vi "Maximize Window.vi"(8 "error in (no error)":errorcluster, 10 "window name (\"\")":string, 11 "window refnum (NaWR)":T1) -> (0 "error out":errorcluster, 3 "window refnum out":T1)   [LabVIEW 2020, in "MacroAssert.lvlib" / "WINUTIL.lvlib"]
doc: "This function will maximize the window named in the window name input, or identified by the window refnum. If an invalid window refnum is passed in, then the function will use the window name to get a window window refnum. If the window cannot be found, an error will be returned."
uses:
  WINUTIL.lvlib
  Window Refnum.ctl
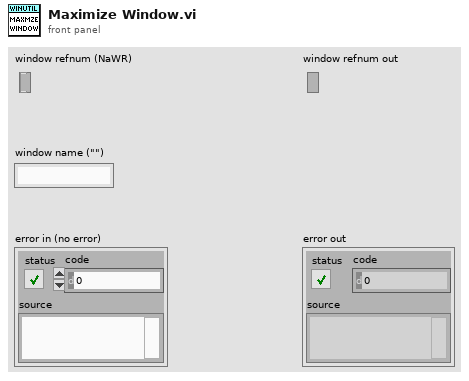
[diagram p1: front panel]
types:
  T1 = typedef "MacroAssert.lvlib/WINUTIL.lvlib/Window Refnum.ctl" = refnum<k1>
  T2 = enum8{"Maximize Window", "Minimize Window", "Show Task List", "Start Screen Saver", "Quit Application"}
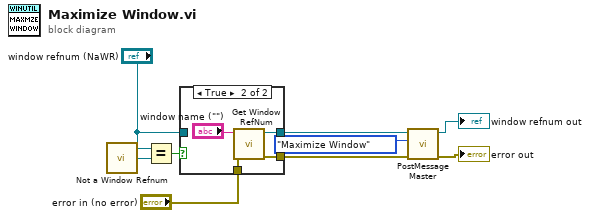
[diagram p0: block diagram]
diagram:
  n1 = call "Not a Window Refnum.vi"() -> ("Not a Window Refnum"=w7:T1)
  n2 = Equal?(x="window refnum (NaWR)", y=w7) -> (x = y?=w8:bool)
  n3 = case shown="True" w8 {
    tunnel: "error in (no error)" -> [w10 w15]
    tunnel: [w11 w14] -> w4
    tunnel: "window refnum (NaWR)" -> [w11 _]
    tunnel: [w10 w13] -> w3
    frame False {
    }
    frame True {
      n4 = call "Get Window RefNum.vi"("error in (no error)"=w15, "window name (\"\")"="window name (\"\")") -> ("error out"=w13:errorcluster, "window refnum (NaWR)"=w14:T1)  [unwired: 8 in]
    }
  }
  n5 = call "PostMessage Master.vi"("error in (no error)"=w3, "function"=T2."Maximize Window", "window refnum"=w4) -> ("error out"=→"error out":errorcluster, "dup window refnum"=→"window refnum out":T1)  [unwired: 7 in]
